vi "CAEN_HVSystem.contents.vi"   [LabVIEW 2014, in "CAEN_HVSystem.lvlib"]
uses:
  CAEN_HVSystem.lvlib
panel:
  # "Refer to blockdiagramm for content VIs."
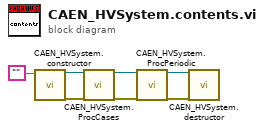
[diagram p0: block diagram]
diagram:
  n1 = call "CAEN_HVSystem.constructor.vi"("name"="") -> ("i ref out"=w6:refnum<vi>, "error out"=w5:errorcluster)  [unwired: 16 in, 1 out]
  n2 = call "CAEN_HVSystem.ProcCases.vi"("i ref in"=w6, "error in (no error)"=w5) -> ("i ref out"=w4:refnum<vi>, "error out"=w3:errorcluster)  [unwired: 15 in, 1 out]
  n3 = call "CAEN_HVSystem.ProcPeriodic.vi"("i ref in"=w4, "error in (no error)"=w3) -> ("i ref out"=w2:refnum<vi>, "error out"=w1:errorcluster)  [unwired: 15 in, 1 out]
  n4 = call "CAEN_HVSystem.destructor.vi"("i ref in"=w2, "error in(no error)"=w1) -> ()  [unwired: 17 in, 1 out]
